vi "FTW-ActorContext-SendMessage.vi"(0 "Actor Reference Prototype":refnum<class "FTW-Actor-Context.lvclass">, 5 "FTW Actor Address":refnum<class "FTW-Actor-Address.lvclass">, 7 "Message":string, 9 "Body":variant, 11 "error in":errorcluster) -> (4 "Actor Reference":refnum<class "FTW-Actor-Context.lvclass">, 6 "FTW Actor Address out":refnum<class "FTW-Actor-Address.lvclass">, 15 "error out":errorcluster)   [LabVIEW 2014, in "FTW-Actor-Context.lvclass"]
uses:
  FTW-Actor-Context.lvclass
  Messaging/Address/FTW-Actor-Address.lvclass
panel:
  # "Inputs"
  # "Outputs"
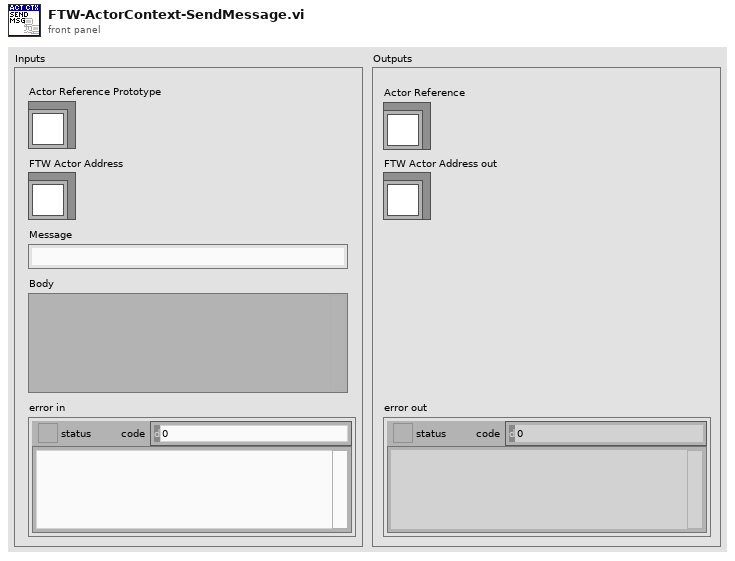
[diagram p1: front panel]
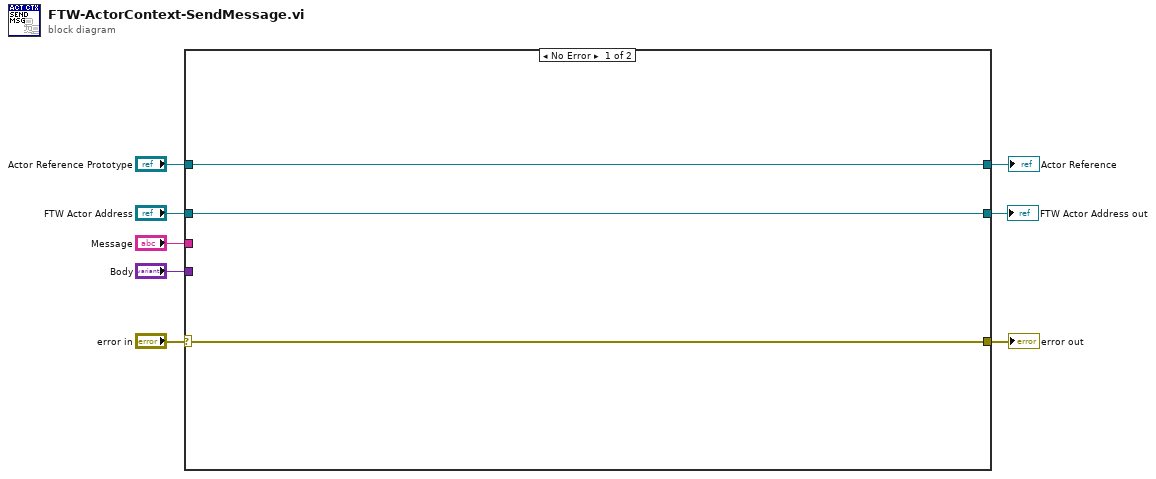
[diagram p0: block diagram]
diagram:
  n1 = case shown="No Error" "error in" {
    selector: "error in" -> [w10 w14]
    tunnel: [w10 w14] -> w8
    tunnel: [w11 w13] -> w6
    tunnel: "Actor Reference Prototype" -> [w11 w13]
    tunnel: [w9 w12] -> w4
    tunnel: "FTW Actor Address" -> [w9 w12]
    tunnel: "Message" -> [_ _]
    tunnel: "Body" -> [_ _]
    frame No Error {
    }
    frame Error {
    }
  }
  "error out" <- w8
  "Actor Reference" <- w6
  "FTW Actor Address out" <- w4
